vi "Open Client Handle.vi"(8 "error in (no error)":errorcluster, 9 "Headers":cluster{"header":string, "value":string}[](array[cluster]), 10 "Request URI":string, 11 "OAuthClient in":refnum<class "OAuthClient.lvclass">) -> (0 "error out":errorcluster, 3 "OAuthClient out":refnum<class "OAuthClient.lvclass">)   [LabVIEW 2020, in "OAuthClient.lvclass"]
uses:
  OAuthClient.lvclass
  OAuthClient.lvclass/OAuthClient.ctl
  <vilib>/LabVIEW Open Source Project/OpenURI/openURI.lvlib
  <vilib>/httpClient/LabVIEWHTTPClient.lvlib
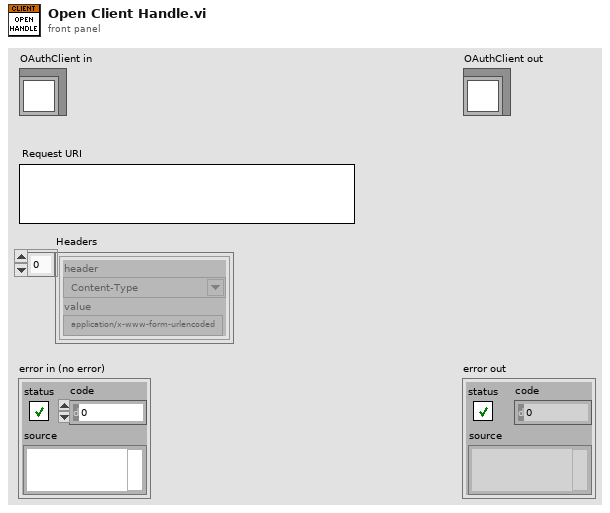
[diagram p1: front panel]
types:
  T1 = typedef "LabVIEWHTTPClient.lvlib/ClientHandle.ctl" = refnum<k1>
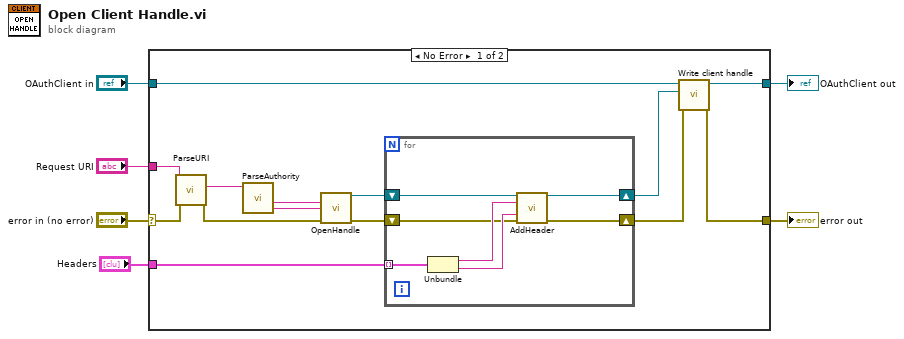
[diagram p0: block diagram]
diagram:
  n1 = case shown="No Error" "error in (no error)" {
    selector: "error in (no error)" -> [w13 w29]
    tunnel: [w12 w29] -> w5
    tunnel: [w19 w28] -> w3
    tunnel: "OAuthClient in" -> [w20 w28]
    tunnel: "Request URI" -> [w18 _]
    tunnel: "Headers" -> [w7 _]
    frame No Error {
      n2 = call <vilib>:"ParseURI.vi"("error in"=w13, "URI"=w18) -> ("error out"=w14:errorcluster, "authority"=w17:string)  [unwired: 4 in, 4 out]
      n3 = call <vilib>:"ParseAuthority.vi"("authority"=w17) -> ("password"=w15:string, "username"=w16:string)  [unwired: 7 in, 2 out]
      n4 = call <vilib>:"OpenHandle.vi"("username"=w16, "password"=w15, "error in (no error)"=w14) -> ("client handle out"=w11:T1, "error out"=w10:errorcluster)  [unwired: 11 in]
      n5 = for {
        shift-right: [w21] -> w9
        shift-left: w11 -> [w26]
        shift-right: [w22] -> w8
        shift-left: w10 -> [w23]
        tunnel: w7 -> [w27] mode=indexing
        n6 = Unbundle(w27) -> ("header"=w25:string, "value"=w24:string)
        n7 = call <vilib>:"AddHeader.vi"("client handle"=w26, "header"=w25, "value"=w24, "error in (no error)"=w23) -> ("client handle out"=w21:T1, "error out"=w22:errorcluster)  [unwired: 10 in]
      }
      n8 = call "Write client handle.vi"("error in (no error)"=w8, "Client Handle"=w9, "OAuthClient in"=w20) -> ("error out"=w12:errorcluster, "OAuthClient out"=w19:refnum<class "OAuthClient.lvclass">)  [unwired: 7 in]
    }
    frame Error {
    }
  }
  "error out" <- w5
  "OAuthClient out" <- w3
